vi "Read Signal Generator Amplitude.vi"(8 "error in (no error)":errorcluster, 11 "PulseData in":refnum<class "PulseData.lvclass">) -> (0 "error out":errorcluster, 2 "Signal Generator Amplitude":dbl, 3 "PulseData out":refnum<class "PulseData.lvclass">)   [LabVIEW 2013, in "Controls Log Monitor.lvlib" / "PulseData.lvclass"]
uses:
  PulseData.lvclass
  PulseData.lvclass/PulseData.ctl
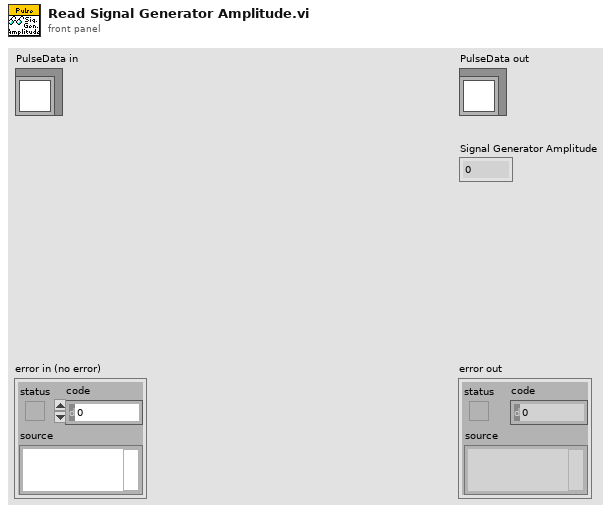
[diagram p1: front panel]
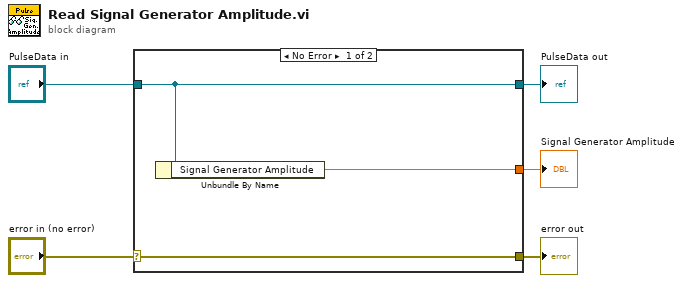
[diagram p0: block diagram]
diagram:
  n1 = case shown="No Error" "error in (no error)" {
    selector: "error in (no error)" -> [w8 w9]
    tunnel: [w8 w9] -> w4
    tunnel: [w7 w10] -> w2
    tunnel: "PulseData in" -> [w7 w10]
    tunnel: [w6 _] -> w1
    frame No Error {
      n2 = Unbundle By Name(w7) -> ("Signal Generator Amplitude"=w6:dbl)
    }
    frame Error {
    }
  }
  "error out" <- w4
  "PulseData out" <- w2
  "Signal Generator Amplitude" <- w1
